vi "WaitRS232.vi"(2 "error in":errorcluster, 3 "delay[160 ms]":u32=160) -> (0 "error out":errorcluster)   [LabVIEW 2017]
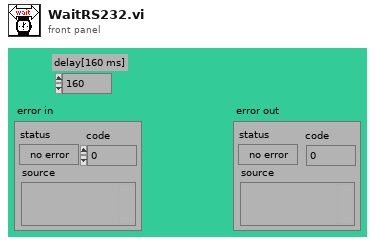
[diagram p1: front panel]
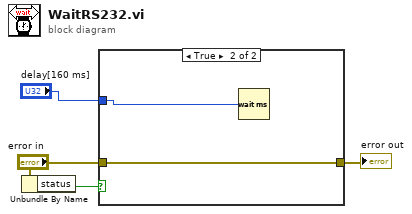
[diagram p0: block diagram]
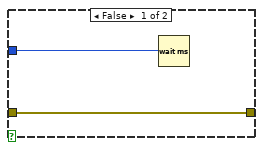
[diagram p2: hidden frame]
diagram:
  n1 = Unbundle By Name("error in") -> ("status"=w3:bool)
  n2 = case shown="True" w3 {
    tunnel: "error in" -> [w6 w8]
    tunnel: [w6 w8] -> w2
    tunnel: "delay[160 ms]" -> [w5 w7]
    frame False {
      n3 = Wait (ms)(milliseconds to wait=w5) -> ()  [unwired: 1 out]
    }
    frame True {
      n4 = Wait (ms)(milliseconds to wait=w7) -> ()  [unwired: 1 out]
    }
  }
  "error out" <- w2
